vi "USRP Packet Transmitter.vi"() -> ()   [LabVIEW 2015]
uses:
  PSD.ctl
  FSK_parameter.ctl
  <vilib>/measure/maspectr.llb/Power Spectrum and PSD Export Mode.ctl
  <instrlib>/niUSRP/niUSRP Write Tx Data (CDB Cluster).vi
  <vilib>/addons/Modulation/Digital/General/MT Generate FSK System Parameters(M).vi
  <vilib>/addons/Modulation/Digital/General/MT Generate PSK System Parameters(M).vi
  <vilib>/addons/Modulation/niDMT.lvlib
  <vilib>/measure/NI_MAPro.lvlib
panel:
  out "Generating?":bool
  out "Symbol Rate [symbols/sec]":dbl=25000.0 format="%#.6p"
  out "Signal Bandwidth[Hz]":dbl format="%#.2p"
  out "FSK Deviation[Hz]":dbl format="%#.2p"
  in  "export mode":T1 caption="导出模式" items=["功率谱", "功率谱密度"]
  out "power spectrum":cluster{"f0":dbl, "df":dbl, "magnitude":dbl[]}(graph)={"f0"=-99999.99999999999, "df"=9.784735812133071, "magnitude"=array[20440 elements]} caption="Power Spectrum"
  in  "autoscale":bool
  out "Constellation Graph":T2(graph)
  in  "stop":bool
  in  "Tab Control":T3=enum."Tx Parameters"
  in  "Message Text":string="Two roads diverged in a yellow wood,\nAnd sorry I could not travel both\nAnd be one traveler, long I stood\nAnd looked down one as far as I could\nTo where it bent in the undergrowth.\n\nThen took the other, as just as fair,\nAnd having perhaps the better claim,\nBecause it was grassy and wanted wear;\nThough as for that the passing there\nHad worn them really about the same.\n\nAnd both that morning equally lay\nIn leaves no step had trodden black.\nOh, I kept the first for another day!\nYet knowing how way leads on to way,\nI doubted if I should ever come back.\n\nI shall be telling this with a sigh\nSomewhere ages and ages hence:\nTwo roads diverged in a wood, and I--\nI took the one less traveled by,\nAnd that has made all the difference.\n"
  in  "Packet Parameters":T4={"Guard Bits "=30, "Sync Bits"=20, "Message Bits"=128}
  in  "Packet Pad \n[samples]":i32=200
  in  "Blank Frame \n[samples]":i32=500
  out "Number of Packets in Message":i32=46
  in  "PN sequence order\nfor Sync Bits":i32=31 caption="PN sequence order (9)"
  in  "Packet Repeat":i32=2
  in  "Pulse Shaping Filter Parameters":T5={"Alpha"=0.5, "Filter Length"=6, "TX Filter"=enum."Root Raised Cos"} caption="Pulse Shaping Filter" {"Alpha" format="%.2f"}
  in  "Tx Parameters":T6={"Tx IQ Sampling\nRate [s/sec]"=500000.0, "Tx Frequency [Hz]"=900000000.0, "Tx Gain [dB]"=0.0, "Tx Antenna"="TX1"} {"Tx Gain [dB]" format="%#.6p"; "Tx Frequency [Hz]" format="%#.6p"; "Tx IQ Sampling\nRate [s/sec]" format="%#.6p"}
  in  "USRP IP address":refnum<k15>="192.168.10.2"
  in  "Modulation  Type":enum32{"PSK", "FSK"}(tab)=enum."FSK"
  in  "Select PSK Modulation Format":T7(tab)=enum."QPSK" caption="PSK"
  in  "BPSK System Parameters":T8={"Samples per Symbol"=8, "symbol map"=[], "Differential PSK"=enum."disable", "PSK type"=0} {"PSK type" items=["normal", "shifted", "offset"]; "symbol map" format="%.3f"}
  in  "QPSK System Parameters":T8={"Samples per Symbol"=8, "symbol map"=[], "Differential PSK"=enum."disable", "PSK type"=0} {"PSK type" items=["normal", "shifted", "offset"]; "symbol map" format="%.3f"}
  in  "pi/4 DQPSK System Parameters":T8={"Samples per Symbol"=8, "symbol map"=[], "Differential PSK"=enum."enable", "PSK type"=1} {"PSK type" items=["normal", "shifted", "offset"]; "symbol map" format="%.3f"}
  in  "OQPSK System Parameters":T8={"Samples per Symbol"=8, "symbol map"=[], "Differential PSK"=enum."disable", "PSK type"=2} {"PSK type" items=["normal", "shifted", "offset"]; "symbol map" format="%.3f"}
  in  "8-PSK System Parameters":T8={"Samples per Symbol"=8, "symbol map"=[], "Differential PSK"=enum."disable", "PSK type"=0} {"PSK type" items=["normal", "shifted", "offset"]; "symbol map" format="%.3f"}
  in  "16-PSK System Parameters":T8={"Samples per Symbol"=8, "symbol map"=[], "Differential PSK"=enum."disable", "PSK type"=0} {"PSK type" items=["normal", "shifted", "offset"]; "symbol map" format="%.3f"}
  in  "M":i32=4 min=2 step=2
  in  "Custom System Parameters":T8={"Samples per Symbol"=8, "symbol map"=[], "Differential PSK"=enum."disable", "PSK type"=0} {"PSK type" items=["normal", "shifted", "offset"]; "symbol map" format="%.3f"}
  in  "MFSK System Parameters":T9={"Samples per Symbol"=16, "symbol map"=[], "M-FSK"=2.0, "FSK Deviation"=50000.0} caption="M-FSK System Parameters" {"FSK Deviation" format="%#_6p"; "symbol map" format="%.3f"}
  out "?":T10 {"?"."Tx IQ Sampling\nRate [s/sec]" format="%#.4p"; "?"."Tx Frequency [Hz]" format="%#.4p"; "?"."Tx Gain [dB]" format="%#.4p"; "Symbol Rate\n [symbols/sec]" format="%#.4p"; "Signal Bandwidth[Hz]" format="%#.4p"; "FSK Deviation[Hz]" format="%#.4p"}
  out "error out":errorcluster
  in  "Queue Length":i32=10
  # "Packet Transmitter--PSK/FSK"
  # "Version: V1.0\nDate: 2019-08-15\nAuthor: Appleking\nOrginization: BJTU"
  # "Guard\nBand"
  # "Sync\nSeq"
  # "Packet\nNumber"
  # "Pad\nData"
  # "Blank\nFrame"
  # "Data"
  # "1、RF参数设置"
  # "3、参数显示"
  # "2、调制参数设置"
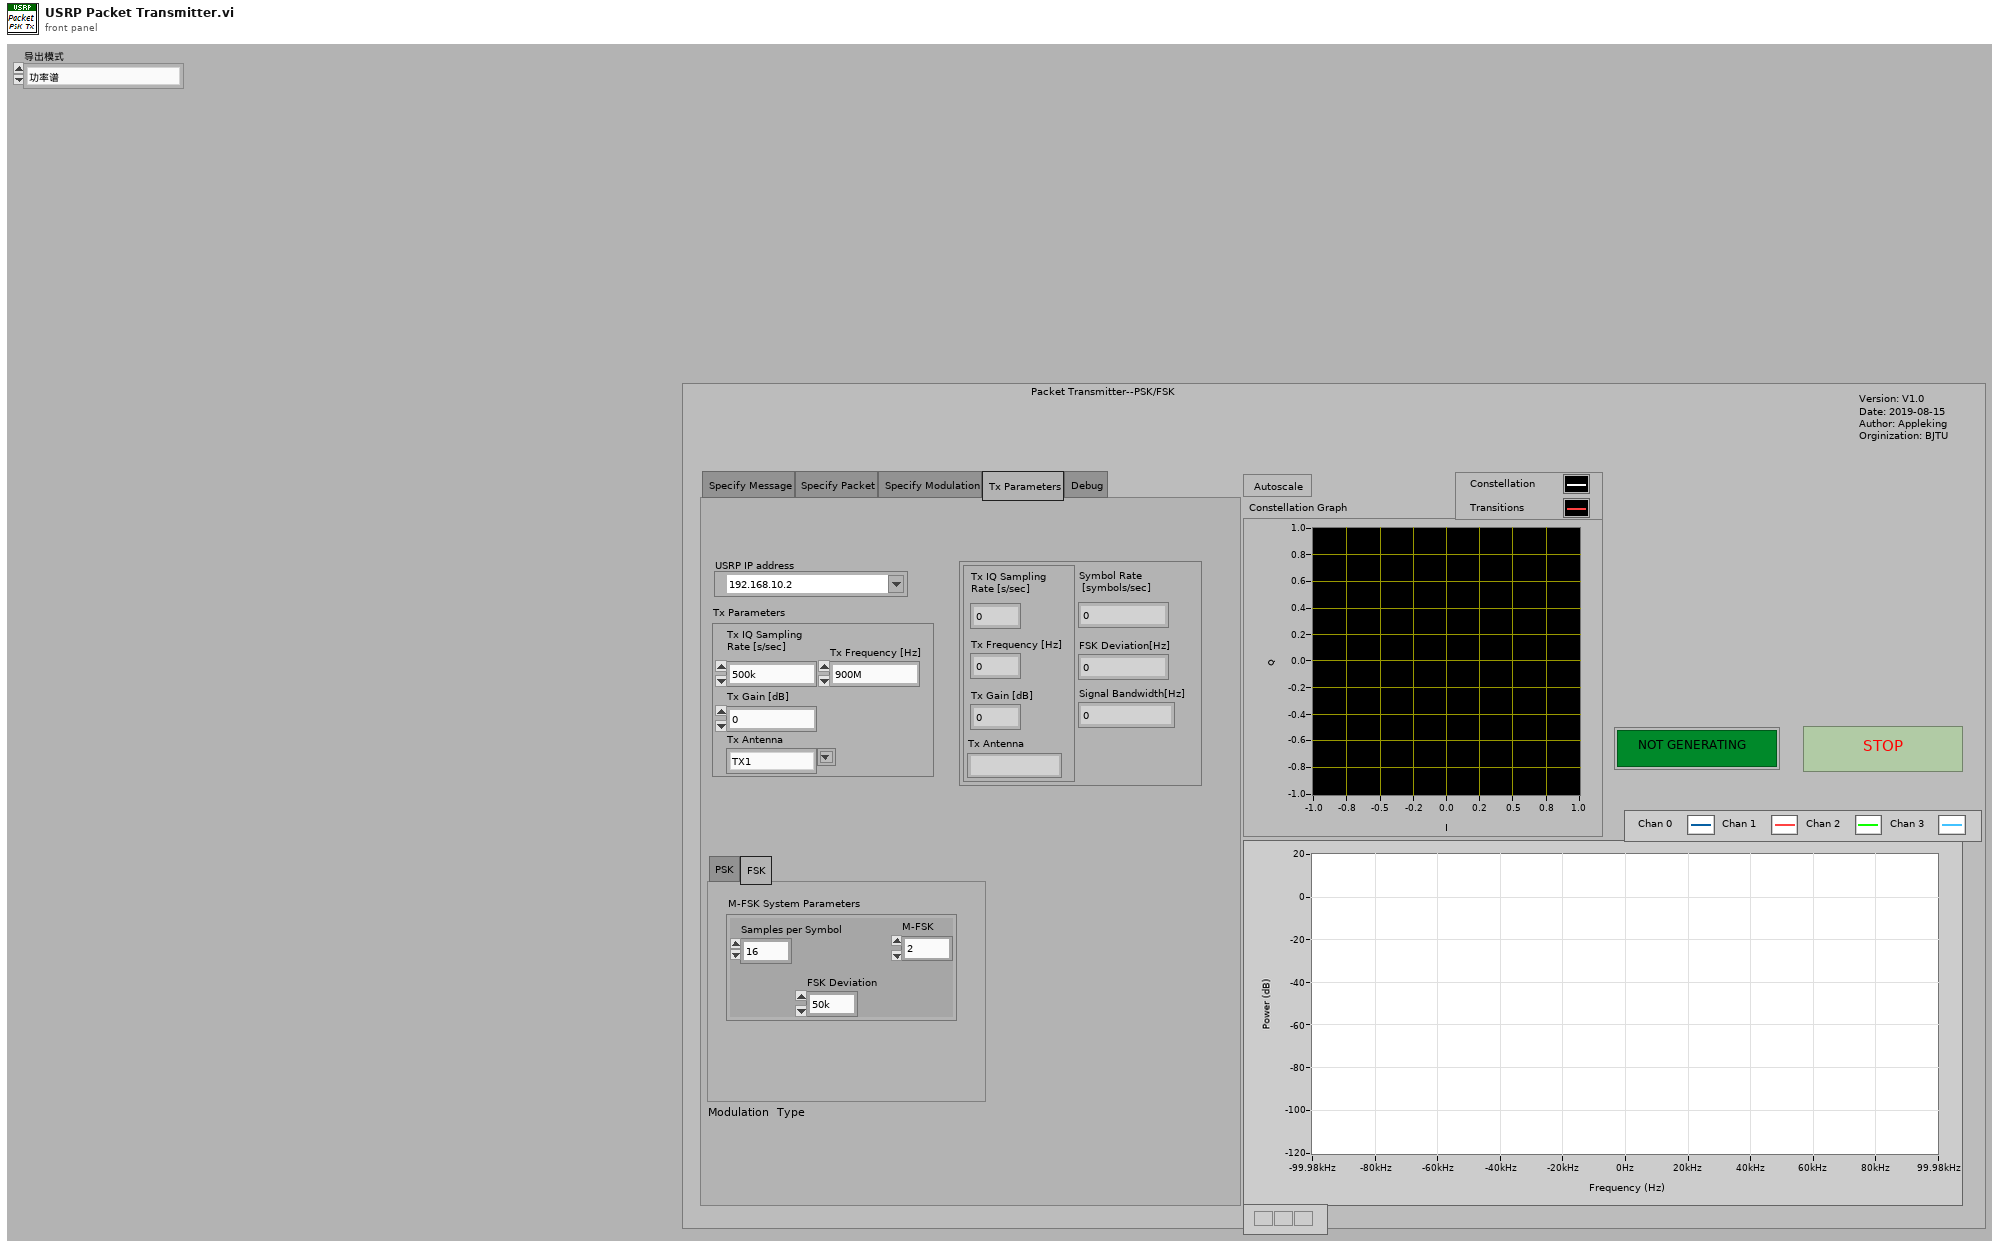
[diagram p1: front panel]
types:
  T1 = typedef "NI_MAPro.lvlib/Power Spectrum and PSD Export Mode.ctl" = u16
  T2 = cluster{"Decimated Array":dbl[], "Decimated Array":dbl[]}[]
  T3 = typedef "PSD.ctl" = enum32{"Specify Message", "Specify Packet", "Specify Modulation", "Tx Parameters", "Debug"}
  T4 = cluster{"Guard Bits ":i32, "Sync Bits":i32, "Message Bits":i32}
  T5 = cluster{"Alpha":dbl, "Filter Length":i32, "TX Filter":enum16{"none", "Raised Cosine", "Root Raised Cos", "Gaussian"}}
  T6 = cluster{"Tx IQ Sampling\nRate [s/sec]":dbl, "Tx Frequency [Hz]":dbl, "Tx Gain [dB]":dbl, "Tx Antenna":string}
  T7 = enum32{"BPSK", "QPSK", "pi/4DQPSK", "OQPSK", "8-PSK", "16-PSK", "Custom"}
  T8 = cluster{"Samples per Symbol":i32, "symbol map":cdb[], "Differential PSK":enum16{"disable", "enable"}, "PSK type":u16}
  T9 = typedef "FSK_parameter.ctl" = cluster{"Samples per Symbol":i32, "symbol map":cdb[], "M-FSK":dbl, "FSK Deviation":dbl}
  T10 = cluster{cluster{"Tx IQ Sampling\nRate [s/sec]":dbl, "Tx Frequency [Hz]":dbl, "Tx Gain [dB]":dbl, "Tx Antenna":string}, "Symbol Rate\n [symbols/sec]":dbl, "Signal Bandwidth[Hz]":dbl, "FSK Deviation[Hz]":dbl}
  T11 = cluster{"samples per symbol (16)":i32, "symbol map":cdb[], "differential PSK":enum16{"disable", "enable"}, "PSK type":u16}
  T12 = cluster{"samples per symbol (16)":i32, "symbol map":dbl[], "symbol phase continuity":enum16{"continuous", "discontinuous"}}
  T13 = cluster{"Actual Tx Parameters":cluster{"Tx IQ Sampling\nRate [s/sec]":dbl, "Tx Frequency [Hz]":dbl, "Tx Gain [dB]":dbl, "Tx Antenna":string}, "Symbol Rate [symbols/sec]":dbl, "Signal Bandwidth[Hz]":dbl, "FSK Deviation[Hz]":dbl}
  T14 = cluster{"s? t:f":cluster{"t0":dbl, "dt":dbl, "Y":cdb[]}, i32}
  T15 = cluster{"output complex waveform":cluster{"t0":dbl, "dt":dbl, "Y":cdb[]}, i32}
  T16 = cluster{"constellation":dbl[], "oversampled data":dbl[]}[]
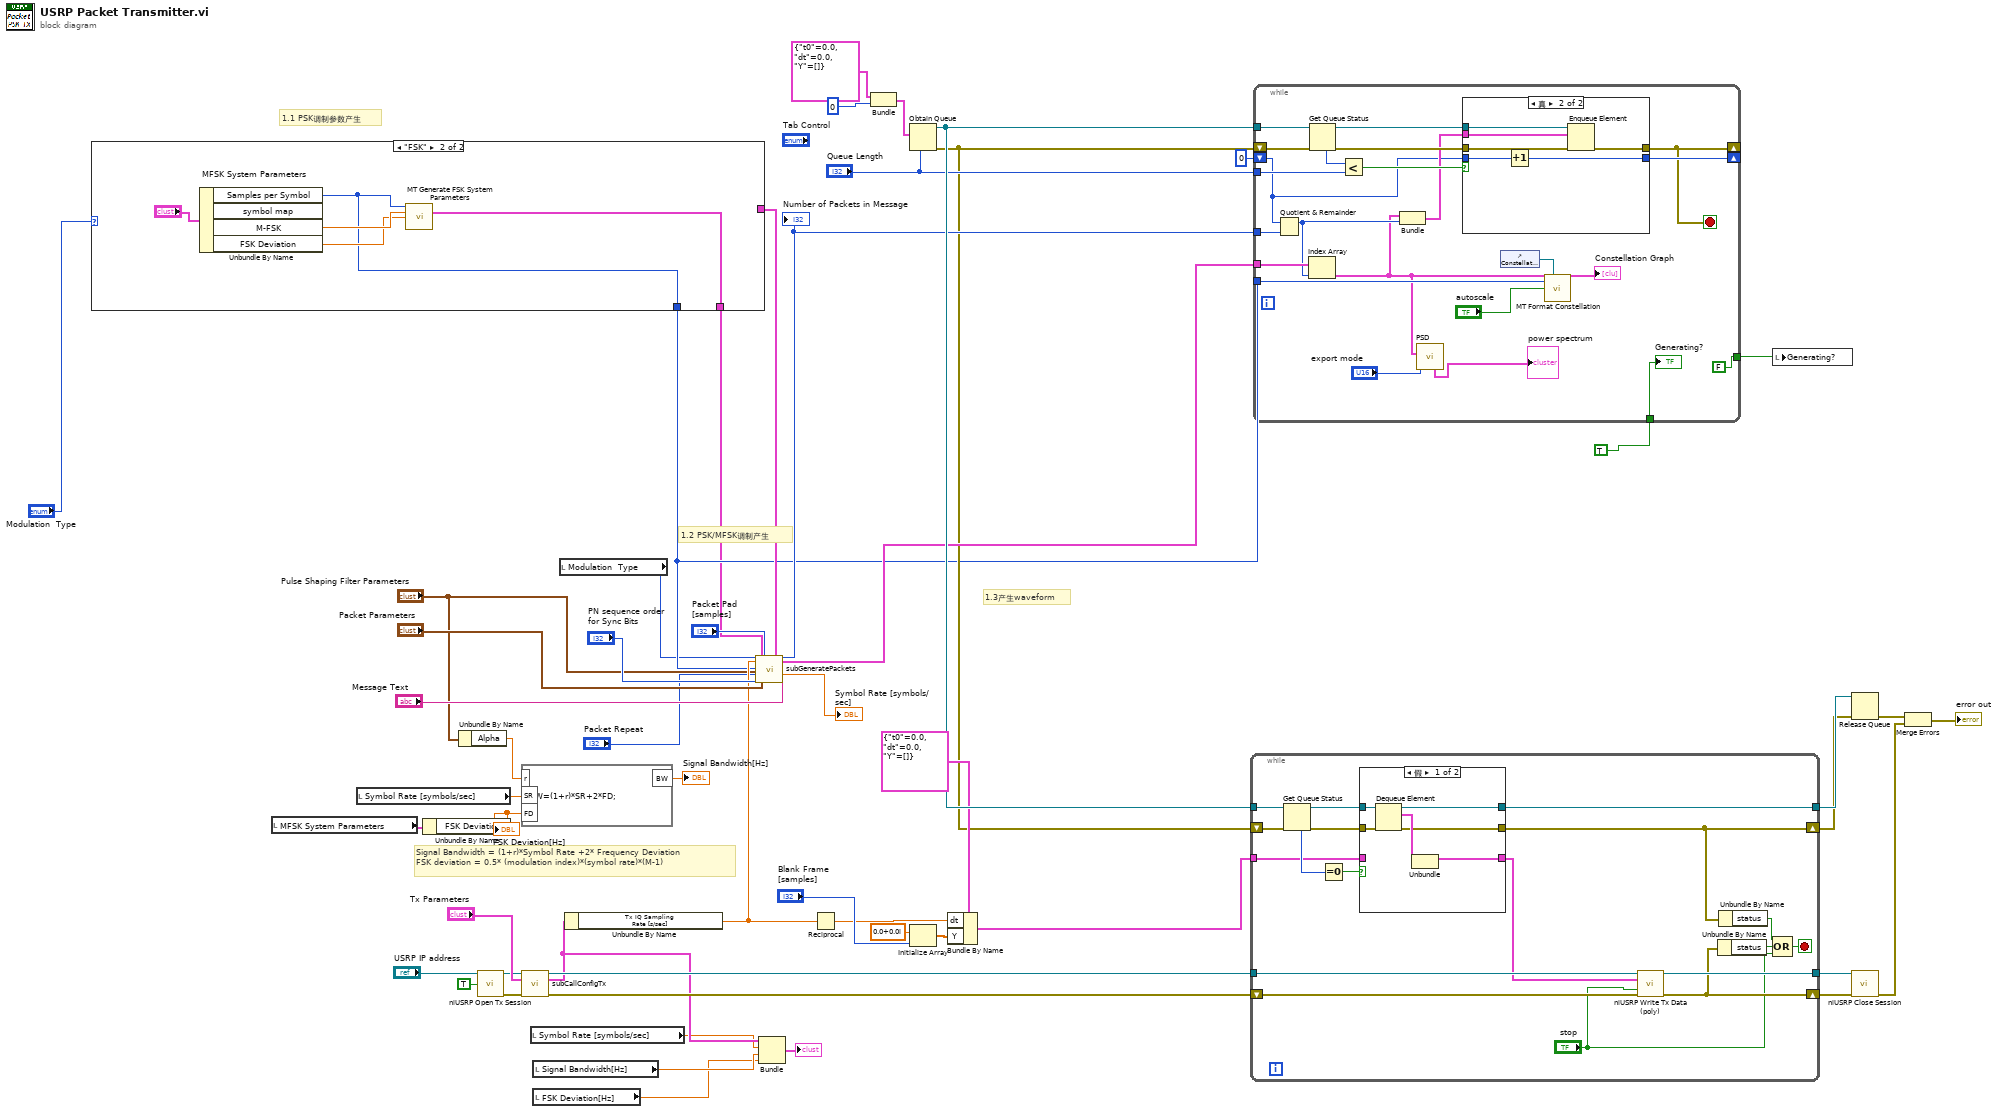
[diagram p0: block diagram]
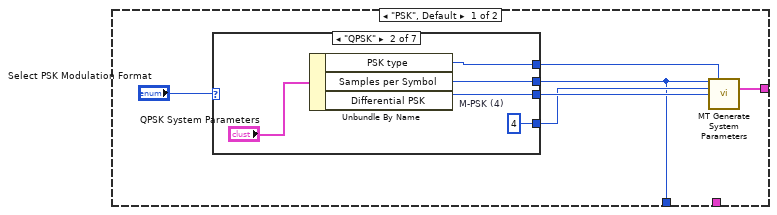
[diagram p2: hidden frame]
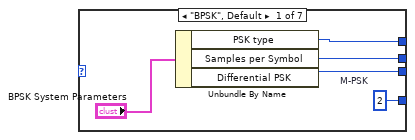
[diagram p3: hidden frame]
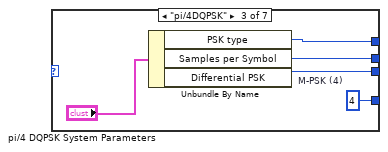
[diagram p4: hidden frame]
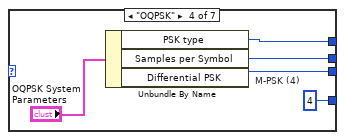
[diagram p5: hidden frame]
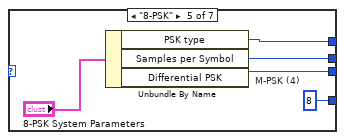
[diagram p6: hidden frame]
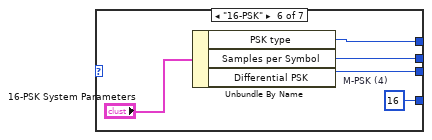
[diagram p7: hidden frame]
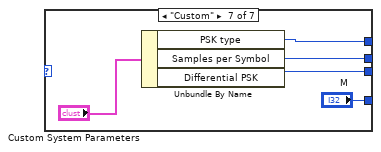
[diagram p8: hidden frame]
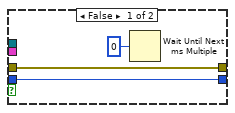
[diagram p9: hidden frame]
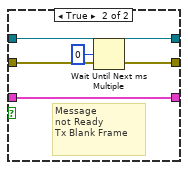
[diagram p10: hidden frame]
diagram:
  # "Signal Bandwidth = (1+r)*Symbol Rate +2* Frequency Deviation\nFSK deviation = 0.5* (modulation index)*(symbol rate)*(M-1)"
  # "1.3产生waveform"
  # "1.2 PSK/MFSK调制产生"
  # "1.1 PSK调制参数产生"
  n1 = case shown="\"FSK\"" "Modulation  Type" {
    tunnel: [w57 _] -> w26
    tunnel: [w55 w96] -> w19
    tunnel: [_ w97] -> w14
    frame "PSK", Default {
      n2 = case shown="\"QPSK\"" "Select PSK Modulation Format" {
        tunnel: [w62 w66 w74 w79 w84 w90 w93] -> w55
        tunnel: [w63 w68 w73 w78 w83 w89 w94] -> w59
        tunnel: [w65 w70 w75 w80 w82 w88 "M"] -> w58
        tunnel: [w64 w69 w72 w77 w85 w87 w95] -> w56
        frame "BPSK", Default {
          w65 = 2  # M-PSK
          n3 = Unbundle By Name("BPSK System Parameters") -> ("PSK type"=w64:u16, "Samples per Symbol"=w62:i32, "Differential PSK"=w63:enum16{"disable", "enable"})
        }
        frame "QPSK" {
          w70 = 4  # M-PSK (4)
          n4 = Unbundle By Name("QPSK System Parameters") -> ("PSK type"=w69:u16, "Samples per Symbol"=w66:i32, "Differential PSK"=w68:enum16{"disable", "enable"})
        }
        frame "pi/4DQPSK" {
          w75 = 4  # M-PSK (4)
          n5 = Unbundle By Name("pi/4 DQPSK System Parameters") -> ("PSK type"=w72:u16, "Samples per Symbol"=w74:i32, "Differential PSK"=w73:enum16{"disable", "enable"})
        }
        frame "OQPSK" {
          w80 = 4  # M-PSK (4)
          n6 = Unbundle By Name("OQPSK System Parameters") -> ("PSK type"=w77:u16, "Samples per Symbol"=w79:i32, "Differential PSK"=w78:enum16{"disable", "enable"})
        }
        frame "8-PSK" {
          w82 = 8  # M-PSK (4)
          n7 = Unbundle By Name("8-PSK System Parameters") -> ("PSK type"=w85:u16, "Samples per Symbol"=w84:i32, "Differential PSK"=w83:enum16{"disable", "enable"})
        }
        frame "16-PSK" {
          w88 = 16  # M-PSK (4)
          n8 = Unbundle By Name("16-PSK System Parameters") -> ("PSK type"=w87:u16, "Samples per Symbol"=w90:i32, "Differential PSK"=w89:enum16{"disable", "enable"})
        }
        frame "Custom" {
          n9 = Unbundle By Name("Custom System Parameters") -> ("PSK type"=w95:u16, "Samples per Symbol"=w93:i32, "Differential PSK"=w94:enum16{"disable", "enable"})
        }
      }
      n10 = call-poly <vilib>:"MT Generate System Parameters.vi"("samples per symbol (16)"=w55, "PSK type"=w56, "M-PSK (4)"=w58, "differential PSK"=w59) -> ("PSK system parameters"=w57:T11)  [unwired: 9 in, 2 out]
    }
    frame "FSK" {
      n11 = Unbundle By Name("MFSK System Parameters") -> ("Samples per Symbol"=w96:i32, "M-FSK"=w99:dbl, "FSK Deviation"=w98:dbl)  [unwired: 1 out]
      n12 = call-poly <vilib>:"MT Generate FSK System Parameters.vi"("samples per symbol (16)"=w96, "M-FSK (2)"=w99, "FSK deviation (Hz)"=w98) -> ("FSK system parameters"=w97:T12)  [unwired: 10 in, 2 out]
    }
  }
  n13 = local read "MFSK System Parameters"() -> (w10:T9)
  n14 = local read "Symbol Rate [symbols/sec]"() -> (w11:dbl)
  n15 = Unbundle By Name(w10) -> ("FSK Deviation"=w9:dbl)
  "FSK Deviation[Hz]" <- w9
  n16 = Unbundle By Name("Pulse Shaping Filter Parameters") -> ("Alpha"=w12:dbl)
  n17 = call <instrlib>:"niUSRP Open Tx Session.vi"("device names"="USRP IP address", "reset"=TRUE) -> ("session handle out"=w29:refnum<k15>, "error out"=w28:errorcluster)  [unwired: 12 in]
  n18 = formula code="BW=(1+r)*SR+2*FD;"("r"=w12, "SR"=w11, "FD"=w9) -> ("BW"=→"Signal Bandwidth[Hz]":dbl)
  n19 = call "subCallConfigTx.vi"("session handle"=w29, "Tx Parameters"="Tx Parameters", "error in"=w28) -> ("session handle out"=w36:refnum<k15>, "Actual Tx Parameters"=w7:T6, "error out"=w41:errorcluster)  [unwired: 10 in]
  n20 = local read "Symbol Rate [symbols/sec]"() -> (w6:dbl)
  n21 = local read "Signal Bandwidth[Hz]"() -> (w5:dbl)
  n22 = local read "FSK Deviation[Hz]"() -> (w4:dbl)
  n23 = local read "Modulation  Type"() -> (w15:enum32{"PSK", "FSK"})
  n24 = Unbundle By Name(w7) -> ("Tx IQ Sampling\nRate [s/sec]"=w20:dbl)
  n25 = call "subGeneratePackets.vi"("调制方式"=w15, "Tx IQ Sampling\nRate [s/sec]"=w20, "Samples per Symbol"=w19, "Pulse Shaping Filter Parameters"="Pulse Shaping Filter Parameters", "Packet Repeat"="Packet Repeat", "PN sequence order\nfor Sync Bits"="PN sequence order\nfor Sync Bits", "FSK system parameters"=w14, "Packet Parameters"="Packet Parameters", "Packet Pad \n[samples]"="Packet Pad \n[samples]", "PSK system parameters"=w26, "Message Text"="Message Text") -> ("Number of Packets"=w35:i32, "Packets"=w43:cluster{"t0":dbl, "dt":dbl, "Y":cdb[]}[], "Symbol Rate"=→"Symbol Rate [symbols/sec]":dbl)  [unwired: 14 in]
  "Number of Packets in Message" <- w35
  n26 = Bundle("Actual Tx Parameters"=w7, "Symbol Rate [symbols/sec]"=w6, "Signal Bandwidth[Hz]"=w5, "FSK Deviation[Hz]"=w4) -> (→"?":T13)  [unwired: 1 in]
  n27 = Reciprocal(x=w20) -> (1/x=w37:dbl)
  n28 = Bundle("s? t:f"=cluster{"t0":dbl, "dt":dbl, "Y":cdb[]} {"t0"=0.0, "dt"=0.0, "Y"=[]}, 0) -> (w46:T14)  [unwired: 1 in]
  n29 = Obtain Queue(max queue size (-1, unlimited)="Queue Length", element data type=w46) -> (queue out=w52:refnum<queue>, error out=w31:errorcluster)  [unwired: 3 in, 1 out]
  n30 = Initialize Array(cdb 0.0+0.0i ("element"), "Blank Frame \n[samples]") -> (w51:cdb[])
  n31 = Bundle By Name(cluster=cluster{"t0":dbl, "dt":dbl, "Y":cdb[]} {"t0"=0.0, "dt"=0.0, "Y"=[]} ("s? t:f"), "dt"=w37, "Y"=w51) -> (w50:cluster{"t0":dbl, "dt":dbl, "Y":cdb[]})
  n32 = while {
    tunnel: w36 -> [w109]
    shift-right: [w106] -> w40
    shift-left: w41 -> [w110]
    tunnel: w52 -> [w118]
    tunnel: w50 -> [w115]
    tunnel: [w114] -> w49
    tunnel: [w108] -> w39
    shift-right: [w103] -> w48
    shift-left: w31 -> [w111]
    stop <- w105 stop-if-true
    n33 = Get Queue Status(queue=w118, error in (no error)=w111) -> (queue out=w113:refnum<queue>, error out=w112:errorcluster, # elements in queue=w117:i32)  [unwired: 1 in, 5 out]
    n34 = Equal To 0?(x=w117) -> (x = 0?=w116:bool)
    n35 = case shown="假" w116 {
      tunnel: w115 -> [_ w128]
      tunnel: [w120 w128] -> w101
      tunnel: [w124 w126] -> w114
      tunnel: [w119 w127] -> w103
      tunnel: w113 -> [w123 w126]
      tunnel: w112 -> [w122 w127]
      frame False {
        n36 = Dequeue Element(queue=w123, error in (no error)=w122) -> (queue out=w124:refnum<queue>, element=w121:T14, error out=w119:errorcluster)  [unwired: 1 in, 1 out]
        n37 = Unbundle(w121) -> ("s? t:f"=w120:cluster{"t0":dbl, "dt":dbl, "Y":cdb[]})  [unwired: 1 out]
      }
      frame True {
        # "Message\nnot Ready\nTx Blank Frame"
        n38 = Wait Until Next ms Multiple(millisecond multiple=u32 0) -> ()  [unwired: 1 out]
      }
    }
    n39 = call-poly <instrlib>:"niUSRP Write Tx Data (poly).vi"("session handle"=w109, "data"=w101, "end of data?"="stop", "error in (no error)"=w110) -> ("session handle out"=w108:refnum<k15>, "error out"=w106:errorcluster)  [unwired: 10 in]
    n40 = Unbundle By Name(w106) -> ("status"=w107:bool)
    n41 = Unbundle By Name(w103) -> ("status"=w102:bool)
    n42 = Compound Arithmetic op=OR(w102, w107, "stop") -> (w105:bool)
  }
  n43 = while {
    tunnel: w52 -> [w151]
    shift-right: [w144] -> _
    shift-left: 0 -> [w140]
    tunnel: w43 -> [w141]
    tunnel: "Queue Length" -> [w143]
    tunnel: w35 -> [w142]
    shift-right: [w138] -> _
    shift-left: w31 -> [w146]
    tunnel: w19 -> [w135]
    tunnel: TRUE -> [w130]
    tunnel: [FALSE] -> w1
    stop <- w138 stop-if-true
    n44 = Quotient & Remainder(x=w140, y=w142) -> (x-y*floor(x/y)=w139:i32)  [unwired: 1 out]
    n45 = Index Array(array=w141, index=w139) -> (element=w131:cluster{"t0":dbl, "dt":dbl, "Y":cdb[]})
    n46 = Get Queue Status(queue=w151, error in (no error)=w146) -> (queue out=w150:refnum<queue>, error out=w147:errorcluster, # elements in queue=w149:i32)  [unwired: 1 in, 5 out]
    n47 = Less?(x=w149, y=w143) -> (x < y?=w148:bool)
    n48 = Bundle("output complex waveform"=w131, w139) -> (w145:T15)  [unwired: 1 in]
    n49 = call "PSD.vi"("output complex waveform"=w131, "export mode"="export mode") -> ("power spectrum"=→"power spectrum":cluster{"f0":dbl, "df":dbl, "magnitude":dbl[]})  [unwired: 8 in, 1 out]
    n50 = case shown="真" w148 {
      tunnel: w147 -> [w152 w160]
      tunnel: w150 -> [_ w159]
      tunnel: [w152 w158] -> w138
      tunnel: w145 -> [_ w157]
      tunnel: w140 -> [w154 w156]
      tunnel: [w154 w155] -> w144
      frame False {
        n51 = Wait Until Next ms Multiple(millisecond multiple=u32 0) -> ()  [unwired: 1 out]
      }
      frame True {
        n52 = Increment(x=w156) -> (x+1=w155:i32)
        n53 = Enqueue Element(queue=w159, element=w157, error in (no error)=w160) -> (error out=w158:errorcluster)  [unwired: 1 in, 2 out]
      }
    }
    n54 = control-ref of="Constellation Graph"() -> (w136:refnum<vi>)
    n55 = call <vilib>:"MT Format Constellation.vi"("waveform"=w131, "constellation reference"=w136, "samples per symbol"=w135, "autoscale"="autoscale") -> ("constellation graph"=→"Constellation Graph":T16)  [unwired: 1 in, 10 out]
    "Generating?" <- w130
  }
  n56 = local write "Generating?"(w1) -> ()
  n57 = Release Queue(queue=w49, error in (no error)=w48) -> (error out=w25:errorcluster)  [unwired: 3 out]
  n58 = call <instrlib>:"niUSRP Close Session.vi"("session handle"=w39, "error in (no error)"=w40) -> ("error out"=w24:errorcluster)  [unwired: 13 in]
  n59 = Merge Errors(w25, w24) -> (→"error out":errorcluster)
